vi "Terminal-GearSystem-Getter20150809.vi"(8 "error in (no error)":errorcluster caption="错误输入（无错误）", 11 "read operation timeout (ms)":i32=5000 caption="读操作超时（5000毫秒）") -> (0 "error out":errorcluster caption="错误输出", 2 "时间标识":timestamp, 3 "设备信息":T1)   [LabVIEW 2014]
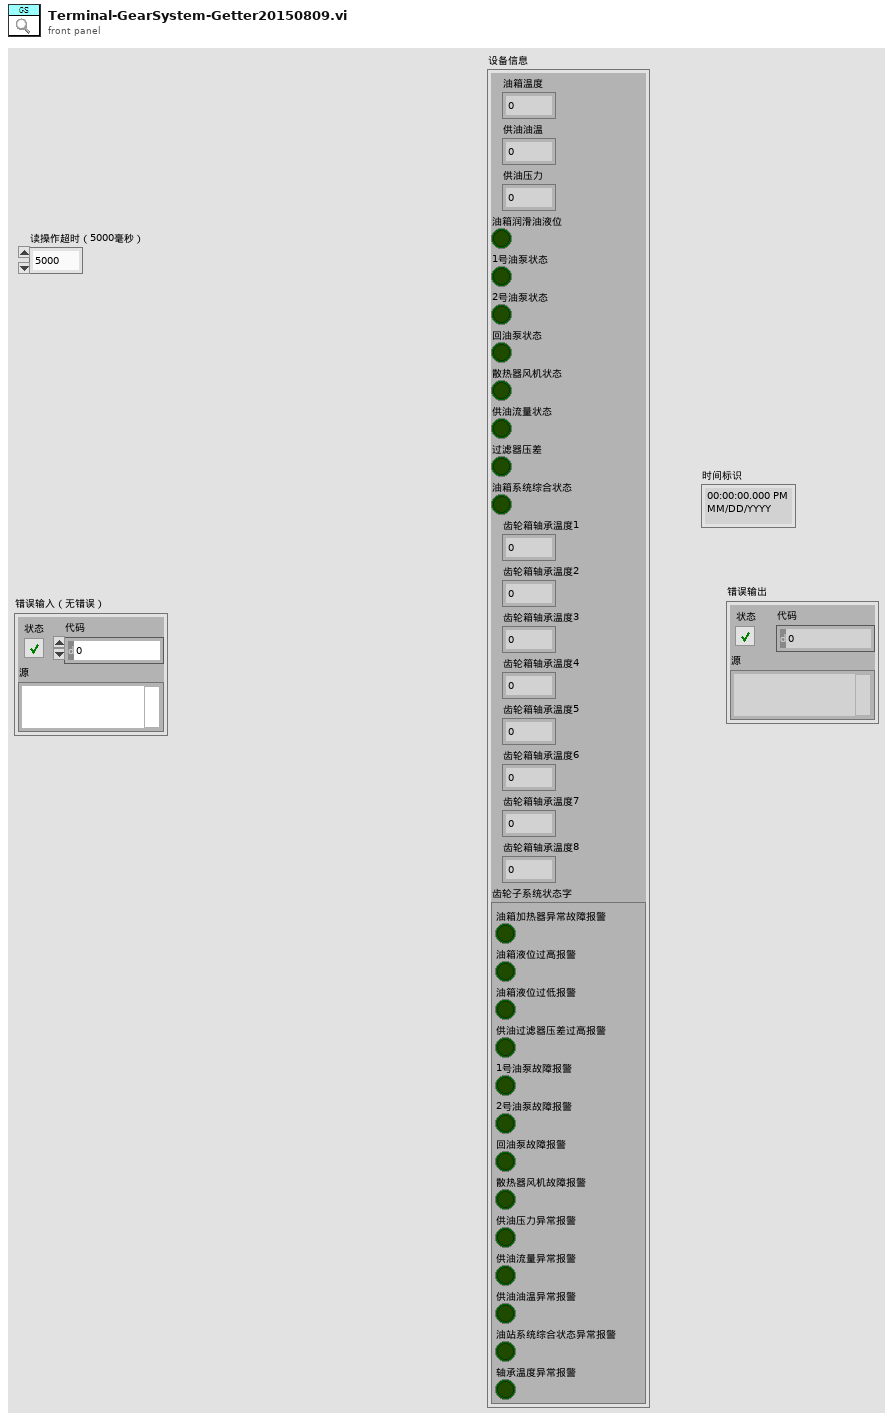
[diagram p1: front panel]
types:
  T1 = cluster{"油箱温度":u16, "供油油温":u16, "供油压力":u16, "油箱润滑油液位":bool, "1号油泵状态":bool, "2号油泵状态":bool, "回油泵状态":bool, "散热器风机状态":bool, "供油流量状态":bool, "过滤器压差":bool, "油箱系统综合状态":bool, "齿轮箱轴承温度1":u16, "齿轮箱轴承温度2":u16, "齿轮箱轴承温度3":u16, "齿轮箱轴承温度4":u16, "齿轮箱轴承温度5":u16, "齿轮箱轴承温度6":u16, "齿轮箱轴承温度7":u16, "齿轮箱轴承温度8":u16, "齿轮子系统状态字":cluster{"油箱加热器异常故障报警":bool, "油箱液位过高报警":bool, "油箱液位过低报警":bool, "供油过滤器压差过高报警":bool, "1号油泵故障报警":bool, "2号油泵故障报警":bool, "回油泵故障报警":bool, "散热器风机故障报警":bool, "供油压力异常报警":bool, "供油流量异常报警":bool, "供油油温异常报警":bool, "油站系统综合状态异常报警":bool, "轴承温度异常报警":bool}}
  T2 = cluster{"油箱温度":u16, "供油油温":u16, "供油压力":u16, "油箱润滑油液位":u16, "1号油泵状态":u16, "2号油泵状态":u16, "回油泵状态":u16, "散热器风机状态":u16, "供油流量状态":u16, "过滤器压差":u16, "油箱系统综合状态":u16, "齿轮箱轴承温度1":u16, "齿轮箱轴承温度2":u16, "齿轮箱轴承温度3":u16, "齿轮箱轴承温度4":u16, "齿轮箱轴承温度5":u16, "齿轮箱轴承温度6":u16, "齿轮箱轴承温度7":u16, "齿轮箱轴承温度8":u16, "齿轮子系统状态字":cluster{"油箱加热器异常故障报警":bool, "油箱液位过高报警":bool, "油箱液位过低报警":bool, "供油过滤器压差过高报警":bool, "1号油泵故障报警":bool, "2号油泵故障报警":bool, "回油泵故障报警":bool, "散热器风机故障报警":bool, "供油压力异常报警":bool, "供油流量异常报警":bool, "供油油温异常报警":bool, "油站系统综合状态异常报警":bool, "轴承温度异常报警":bool}}
  T3 = cluster{"油箱加热器异常故障报警":bool, "油箱液位过高报警":bool, "油箱液位过低报警":bool, "供油过滤器压差过高报警":bool, "1号油泵故障报警":bool, "2号油泵故障报警":bool, "回油泵故障报警":bool, "散热器风机故障报警":bool, "供油压力异常报警":bool, "供油流量异常报警":bool, "供油油温异常报警":bool, "油站系统综合状态异常报警":bool, "轴承温度异常报警":bool}
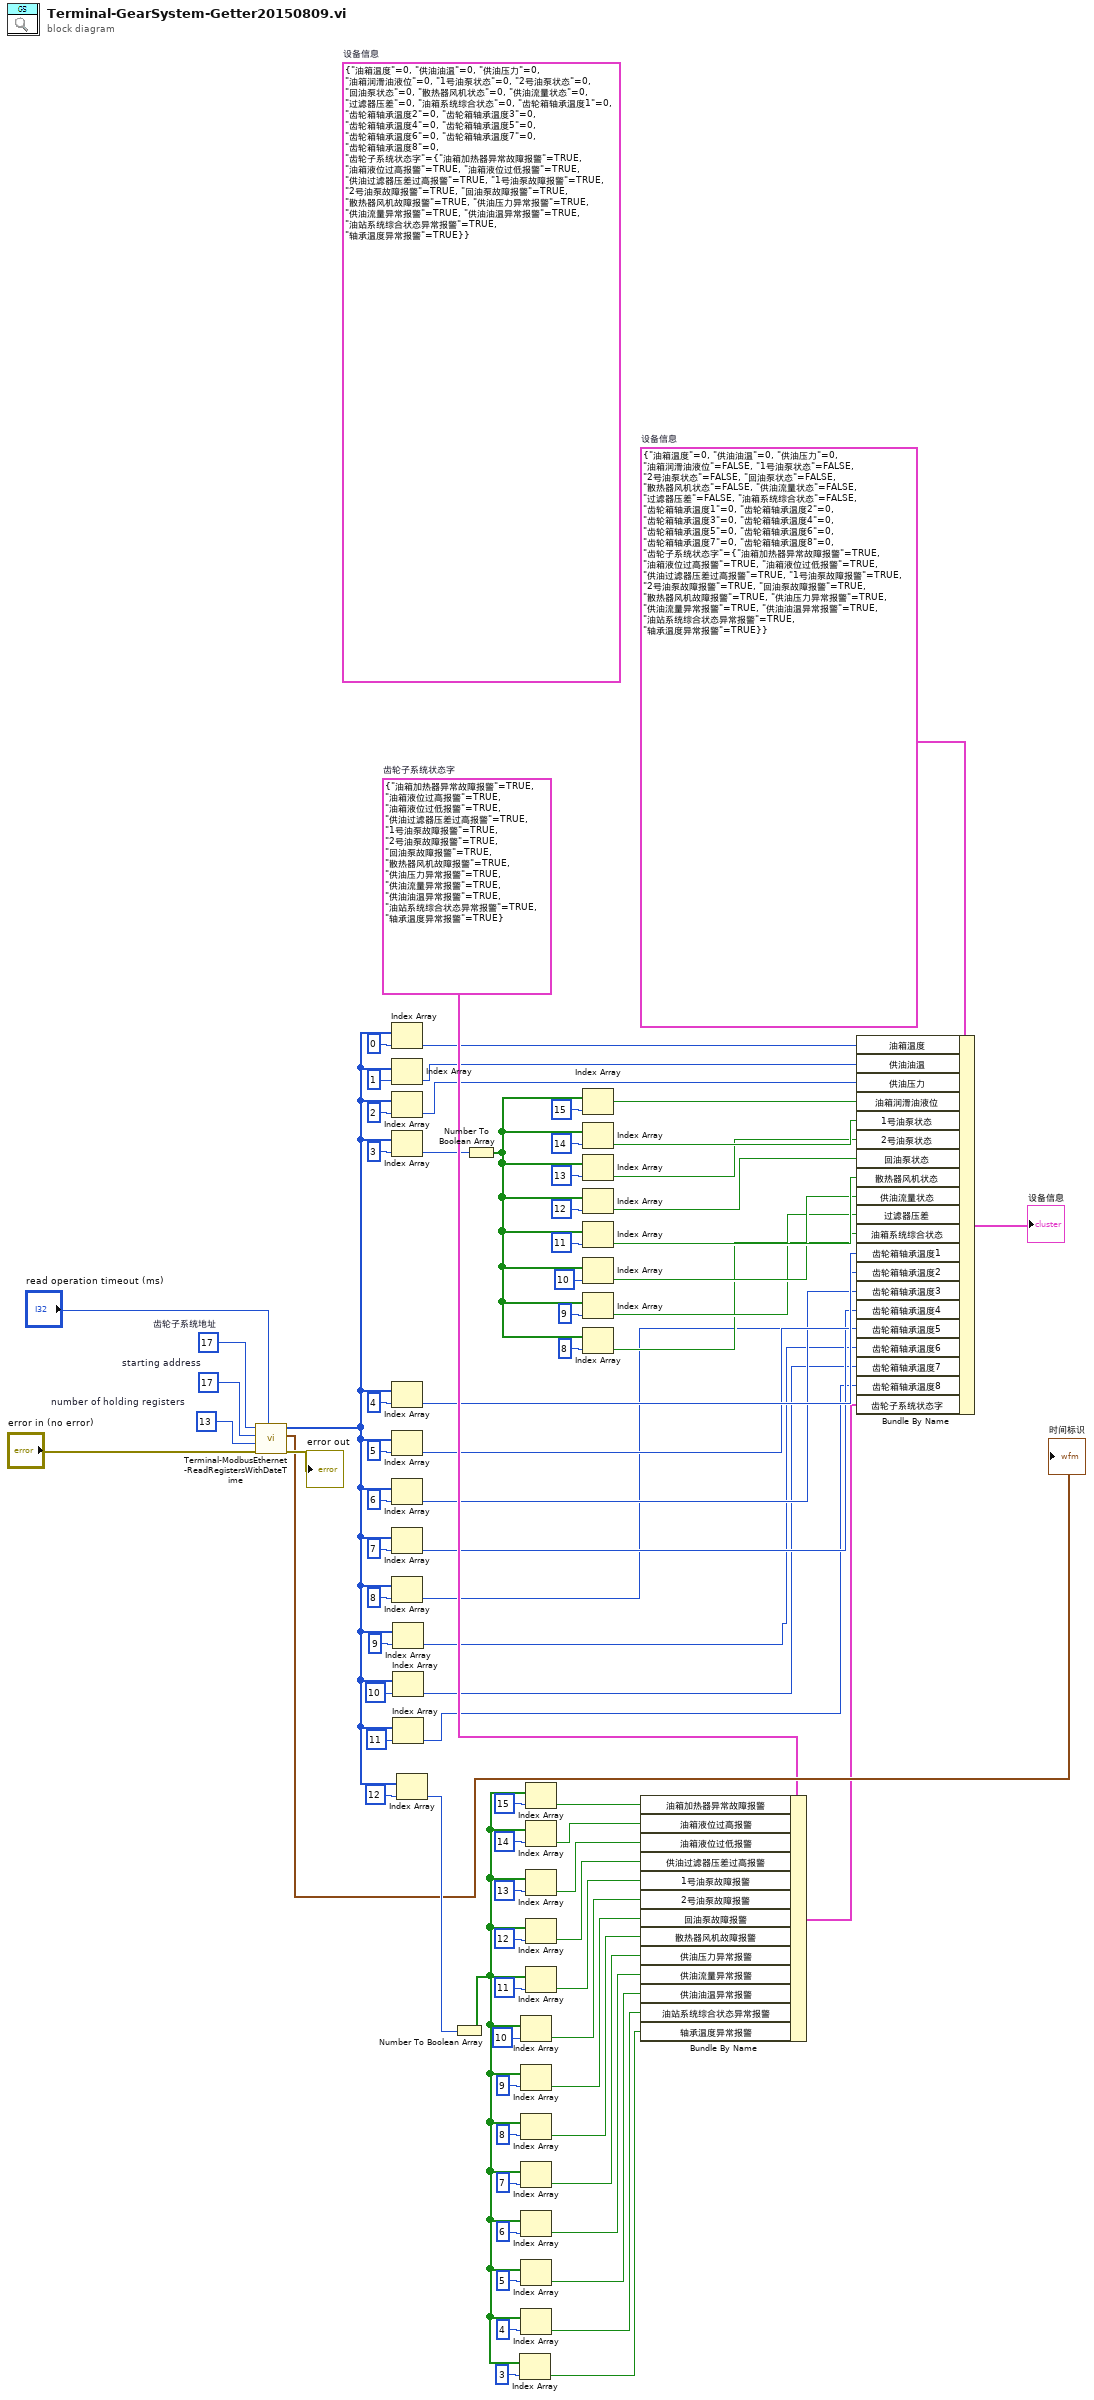
[diagram p0: block diagram]
diagram:
  (unwired) T2 {"油箱温度"=0, "供油油温"=0, "供油压力"=0, "油箱润滑油液位"=0, "1号油泵状态"=0, "2号油泵状态"=0, "回油泵状态"=0, "散热器风机状态"=0, "供油流量状态"=0, "过滤器压差"=0, "油箱系统综合状态"=0, "齿轮箱轴承温度1"=0, "齿轮箱轴承温度2"=0, "齿轮箱轴承温度3"=0, "齿轮箱轴承温度4"=0, "齿轮箱轴承温度5"=0, "齿轮箱轴承温度6"=0, "齿轮箱轴承温度7"=0, "齿轮箱轴承温度8"=0, "齿轮子系统状态字"={"油箱加热器异常故障报警"=TRUE, "油箱液位过高报警"=TRUE, "油箱液位过低报警"=TRUE, "供油过滤器压差过高报警"=TRUE, "1号油泵故障报警"=TRUE, "2号油泵故障报警"=TRUE, "回油泵故障报警"=TRUE, "散热器风机故障报警"=TRUE, "供油压力异常报警"=TRUE, "供油流量异常报警"=TRUE, "供油油温异常报警"=TRUE, "油站系统综合状态异常报警"=TRUE, "轴承温度异常报警"=TRUE}}  # 设备信息
  w39 = T3 {"油箱加热器异常故障报警"=TRUE, "油箱液位过高报警"=TRUE, "油箱液位过低报警"=TRUE, "供油过滤器压差过高报警"=TRUE, "1号油泵故障报警"=TRUE, "2号油泵故障报警"=TRUE, "回油泵故障报警"=TRUE, "散热器风机故障报警"=TRUE, "供油压力异常报警"=TRUE, "供油流量异常报警"=TRUE, "供油油温异常报警"=TRUE, "油站系统综合状态异常报警"=TRUE, "轴承温度异常报警"=TRUE}  # 齿轮子系统状态字
  w76 = T1 {"油箱温度"=0, "供油油温"=0, "供油压力"=0, "油箱润滑油液位"=FALSE, "1号油泵状态"=FALSE, "2号油泵状态"=FALSE, "回油泵状态"=FALSE, "散热器风机状态"=FALSE, "供油流量状态"=FALSE, "过滤器压差"=FALSE, "油箱系统综合状态"=FALSE, "齿轮箱轴承温度1"=0, "齿轮箱轴承温度2"=0, "齿轮箱轴承温度3"=0, "齿轮箱轴承温度4"=0, "齿轮箱轴承温度5"=0, "齿轮箱轴承温度6"=0, "齿轮箱轴承温度7"=0, "齿轮箱轴承温度8"=0, "齿轮子系统状态字"={"油箱加热器异常故障报警"=TRUE, "油箱液位过高报警"=TRUE, "油箱液位过低报警"=TRUE, "供油过滤器压差过高报警"=TRUE, "1号油泵故障报警"=TRUE, "2号油泵故障报警"=TRUE, "回油泵故障报警"=TRUE, "散热器风机故障报警"=TRUE, "供油压力异常报警"=TRUE, "供油流量异常报警"=TRUE, "供油油温异常报警"=TRUE, "油站系统综合状态异常报警"=TRUE, "轴承温度异常报警"=TRUE}}  # 设备信息
  w80 = u16 13  # number of holding registers
  w81 = u16 17  # starting address
  w82 = u8 17  # 齿轮子系统地址
  n1 = call "Terminal-ModbusEthernet-ReadRegistersWithDateTime.vi"("read operation timeout (ms)"="read operation timeout (ms)", "error in"="error in (no error)", "number of holding registers"=w80, "starting address"=w81, "unit ID"=w82) -> ("error out"=→"error out":errorcluster, "时间标识"=→"时间标识":timestamp, "register values"=w14:u16[])  [unwired: 4 in]
  n2 = Index Array(array=w14, index=0 ("索引")) -> (element=w38:u16)
  n3 = Index Array(array=w14, index=1 ("索引")) -> (element=w37:u16)
  n4 = Index Array(array=w14, index=2 ("索引")) -> (element=w36:u16)
  n5 = Index Array(array=w14, index=3 ("索引")) -> (element=w35:u16)
  n6 = Index Array(array=w14, index=4 ("索引")) -> (element=w13:u16)
  n7 = Index Array(array=w14, index=5 ("索引")) -> (element=w12:u16)
  n8 = Index Array(array=w14, index=6 ("索引")) -> (element=w11:u16)
  n9 = Index Array(array=w14, index=7 ("索引")) -> (element=w10:u16)
  n10 = Index Array(array=w14, index=8 ("索引")) -> (element=w9:u16)
  n11 = Index Array(array=w14, index=9 ("索引")) -> (element=w8:u16)
  n12 = Index Array(array=w14, index=10 ("索引")) -> (element=w7:u16)
  n13 = Index Array(array=w14, index=11 ("索引")) -> (element=w6:u16)
  n14 = Index Array(array=w14, index=12 ("索引")) -> (element=w71:u16)
  n15 = Number To Boolean Array(number=w71) -> (Boolean array=w4:bool[])
  n16 = Number To Boolean Array(number=w35) -> (Boolean array=w26:bool[])
  n17 = Index Array(array=w4, index=3 ("索引")) -> (element=w3:bool)
  n18 = Index Array(array=w4, index=10 ("索引")) -> (element=w47:bool)
  n19 = Index Array(array=w4, index=9 ("索引")) -> (element=w46:bool)
  n20 = Index Array(array=w4, index=8 ("索引")) -> (element=w45:bool)
  n21 = Index Array(array=w4, index=7 ("索引")) -> (element=w44:bool)
  n22 = Index Array(array=w4, index=6 ("索引")) -> (element=w41:bool)
  n23 = Index Array(array=w4, index=5 ("索引")) -> (element=w42:bool)
  n24 = Index Array(array=w4, index=4 ("索引")) -> (element=w43:bool)
  n25 = Index Array(array=w4, index=15 ("索引")) -> (element=w67:bool)
  n26 = Index Array(array=w4, index=14 ("索引")) -> (element=w66:bool)
  n27 = Index Array(array=w4, index=13 ("索引")) -> (element=w50:bool)
  n28 = Index Array(array=w4, index=12 ("索引")) -> (element=w49:bool)
  n29 = Index Array(array=w4, index=11 ("索引")) -> (element=w48:bool)
  n30 = Index Array(array=w26, index=15 ("索引")) -> (element=w25:bool)
  n31 = Index Array(array=w26, index=14 ("索引")) -> (element=w24:bool)
  n32 = Index Array(array=w26, index=13 ("索引")) -> (element=w23:bool)
  n33 = Index Array(array=w26, index=12 ("索引")) -> (element=w22:bool)
  n34 = Index Array(array=w26, index=11 ("索引")) -> (element=w21:bool)
  n35 = Index Array(array=w26, index=10 ("索引")) -> (element=w20:bool)
  n36 = Index Array(array=w26, index=9 ("索引")) -> (element=w19:bool)
  n37 = Index Array(array=w26, index=8 ("索引")) -> (element=w18:bool)
  n38 = Bundle By Name(cluster=w39, "油箱加热器异常故障报警"=w67, "油箱液位过高报警"=w66, "油箱液位过低报警"=w50, "供油过滤器压差过高报警"=w49, "1号油泵故障报警"=w48, "2号油泵故障报警"=w47, "回油泵故障报警"=w46, "散热器风机故障报警"=w45, "供油压力异常报警"=w44, "供油流量异常报警"=w41, "供油油温异常报警"=w42, "油站系统综合状态异常报警"=w43, "轴承温度异常报警"=w3) -> (w2:T3)
  n39 = Bundle By Name(cluster=w76, "油箱温度"=w38, "供油油温"=w37, "供油压力"=w36, "油箱润滑油液位"=w25, "1号油泵状态"=w24, "2号油泵状态"=w23, "回油泵状态"=w22, "散热器风机状态"=w21, "供油流量状态"=w20, "过滤器压差"=w19, "油箱系统综合状态"=w18, "齿轮箱轴承温度1"=w13, "齿轮箱轴承温度2"=w12, "齿轮箱轴承温度3"=w11, "齿轮箱轴承温度4"=w10, "齿轮箱轴承温度5"=w9, "齿轮箱轴承温度6"=w8, "齿轮箱轴承温度7"=w7, "齿轮箱轴承温度8"=w6, "齿轮子系统状态字"=w2) -> (→"设备信息":T1)
